vi "Fetch Multiple Points.vi"(8 "error in (no error)":errorcluster, 9 "Timeout (10000 ms)":i32=10000 format="%#.6g", 11 "VISA resource name":refnum<visa-resource-name>) -> (0 "error out":errorcluster, 2 "Measurements":dbl[][](array[numeric]), 3 "VISA resource name out":refnum<visa-resource-name>)   [LabVIEW 2015, in "Template - DMM.lvlib"]
doc: "This low-level VI returns an array of values from a previously initiated measurement. The number of measurements the DMM takes is determined by the values you specify for the <B>Trigger Count</B> control and <B>Sample Count</B> control of the <B>Configure Multipoint</B> VI.\n\n<B>Note:</B> Use this VI only with other low-level VIs. The high-level VIs automatically incorporate this functionality. This VI does not check the instrument status. If you want to check the instrument status, call the <B>Error Query</B> VI at the conclusion of the sequence."
uses:
  <instrlib>/_Template - DMM/Template - DMM.lvlib
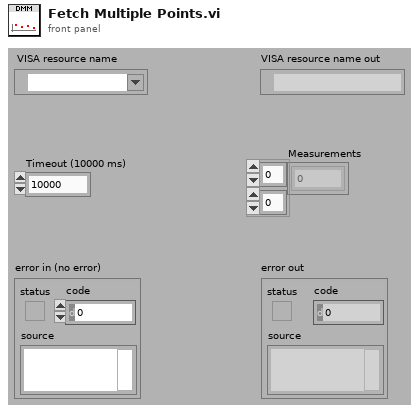
[diagram p1: front panel]
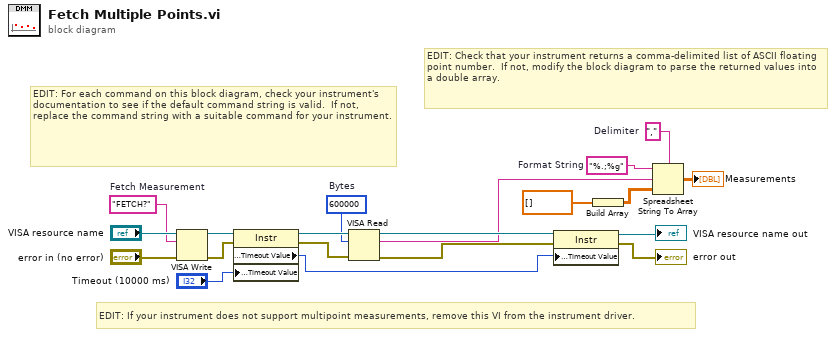
[diagram p0: block diagram]
diagram:
  w16 = ","  # Delimiter
  w17 = "%.;%g"  # Format String
  w18 = "FETCH?"  # Fetch Measurement
  w3 = u32 600000  # Bytes
  # "EDIT: If your instrument does not support multipoint measurements, remove this VI from the instrument driver."
  # "EDIT: Check that your instrument returns a comma-delimited list of ASCII floating point number.  If not, modify the block diagram to parse the returned values into a double array."
  # "EDIT: For each command on this block diagram, check your instrument's documentation to see if the default command string is valid.  If not, replace the command string with a suitable command for your instrument."
  n1 = VISA Write(VISA resource name="VISA resource name", write buffer=w18, error in (no error)="error in (no error)") -> (VISA resource name out=w14:refnum<visa-resource-name>, error out=w13:errorcluster)  [unwired: 1 out]
  n2 = property on="Property Node" class="Instr"(reference=w14, error in=w13, "General Settings:Timeout Value"="Timeout (10000 ms)") -> (reference out=w12:refnum<visa-resource-name>, error out=w11:errorcluster, "General Settings:Timeout Value"=w7:u32)
  n3 = VISA Read(VISA resource name=w12, byte count=w3, error in (no error)=w11) -> (VISA resource name out=w9:refnum<visa-resource-name>, read buffer=w4:string, error out=w8:errorcluster)  [unwired: 1 out]
  n4 = property on="Property Node" class="Instr"(reference=w9, error in=w8, "General Settings:Timeout Value"=w7) -> (reference out=→"VISA resource name out":refnum<visa-resource-name>, error out=→"error out":errorcluster)
  n5 = Build Array(dbl[] []) -> (w15:dbl[][])
  n6 = Spreadsheet String To Array(delimiter (Tab)=w16, format string=w17, spreadsheet string=w4, array type (2D Dbl)=w15) -> (array=→"Measurements":dbl[][])
